vi "client.vi"() -> ()   [LabVIEW 2024]
panel:
  in  "Reset Button":bool
  in  "Historical Log Path":path
  out "Average Temperature (Last 5)":dbl
  in  "Password Input":string
  in  "Heater ON/OFF 2":bool
  out "System Status":enum16{"Automatic", "Manual", "Maintenance"}(ring)
  out "Heater Status":T1(ring)
  in  "Manual/Automatic switch":bool
  in  "Sample rate":dbl
  in  "Temperature setpoint control high":dbl
  in  "Temperature setpoint control low":dbl
  in  "Power ON/OFF 2":bool
  out "Historical temperature reading":dbl[](graph)
  out "Min temperature reading":dbl
  out "Max temperature reading":dbl
  out "Current temperature reading":dbl(slide) scale=0.0..150.0
  out "Heater ON/OFF":bool
  out "Power ON/OFF":bool
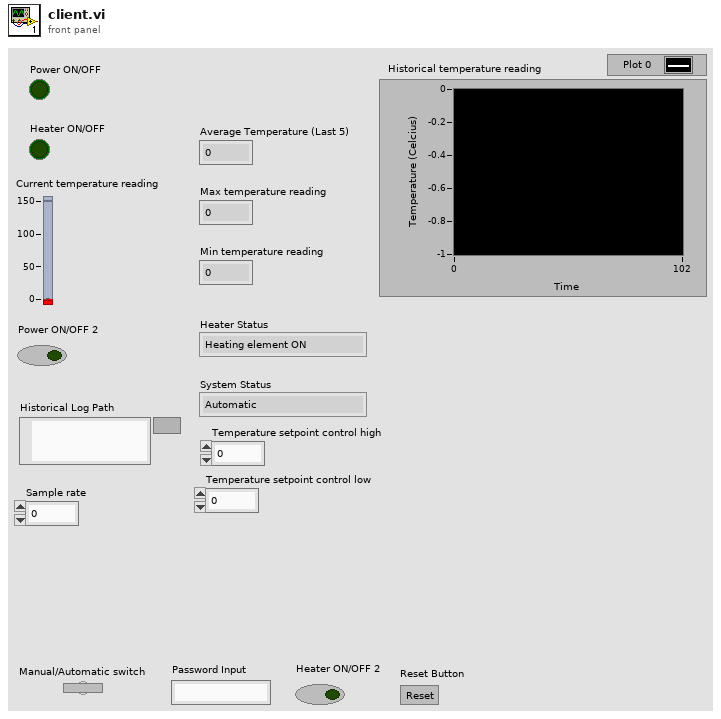
[diagram p1: front panel]
types:
  T1 = enum16{"Heating element ON", "Heating element OFF"}
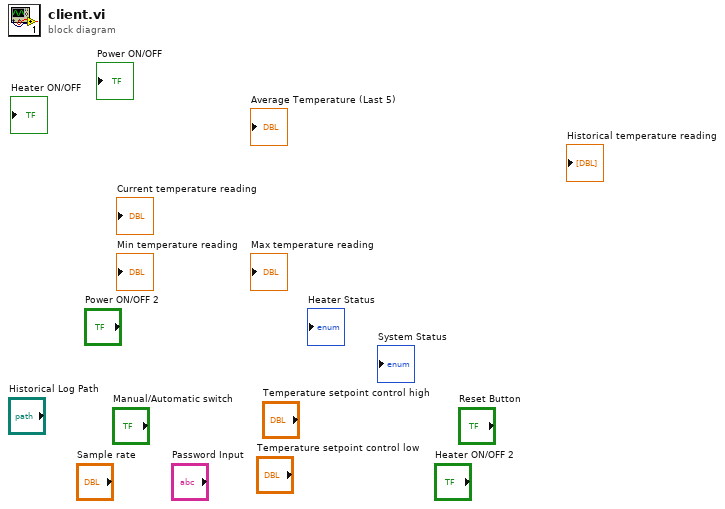
[diagram p0: block diagram]
diagram:
